vi "Suppress Error Code.vi"   [LabVIEW 2020]
doc: "This polymorphic VI takes either an error code or an array of error codes. If the error code being passed in through Error In is either the scalar or in the array of error codes it will not be passed to Error Out. Any other error codes will be passed to Error Out.\n\nFreeware from Moore Good Ideas, www.mooregoodideas.com. Do not remove this line."
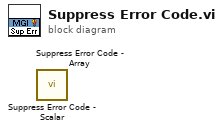
[diagram p0: block diagram]
diagram:
  n1 = call "Suppress Error Code - Scalar.vi"() -> ()  [unwired: 10 in, 2 out]
  n2 = call "Suppress Error Code - Array.vi"() -> ()  [unwired: 10 in, 2 out]
